vi "Agilent 33XXX Series Generate Modulated Waveform.vi"() -> ()   [LabVIEW 2010, in "AWG.lvlib"]
doc: "Shows how to configure and generate an amplitude modulated waveform."
uses:
  AWG.lvlib
  Agilent 33XXX Series.lvlib
  Public/Configure/Configure Modulation (Amplitude).vi
panel:
  in  "Serial Configuration":T1={"Baud Rate"=9600, "Parity"=0, "Data Bits"=8, "Flow Control"=4} {"Flow Control" items=["None", "XON/XOFF", "RTS/CTS", "XON/XOFF & RTS/CTS", "DTR/DSR", "XON/XOFF & DTR/DSR"]; "Data Bits" items=["7"=7, "8"=8]; "Parity" items=["None", "Odd", "Even", "Mark", "Space"]; "Baud Rate" items=["300"=300, "600"=600, "1200"=1200, "2400"=2400, "4800"=4800, "9600"=9600, "19200"=19200]}
  in  "DC Offset (0.00 V)":dbl
  in  "Amplitude (1 Vpp)":dbl=1.0
  in  "Waveform Function (1: Sine)":u16(ring)=1 items=["DC", "Sine", "Square", "Triangle", "Ramp", "Pulse", "Noise", "Sinc", "Negative Ramp", "Exponential Rise", "Exponential Fall", "Cardiac"]
  in  "Frequency (1000 Hz)":dbl=1000.0
  in  "Modulation Waveform (0: Sine)":i32(ring) items=["Sine", "Square", "Ramp", "Negative Ramp", "Triangle", "Noise", "Arbitrary Waveform"]
  in  "Amplitude Modulation Source (0: Internal)":i32(ring) items=["Internal", "External"]
  in  "Modulation Depth (100 %)":i32=100
  in  "Modulation Frequency (1000 Hz)":dbl=1000.0
  in  "VISA resource name":refnum<visa-resource-name>
  # "(c) 2005 - 2013 National Instruments.  ALL RIGHTS RESERVED."
  # "Carrier Settings"
  # "Modulation Settings"
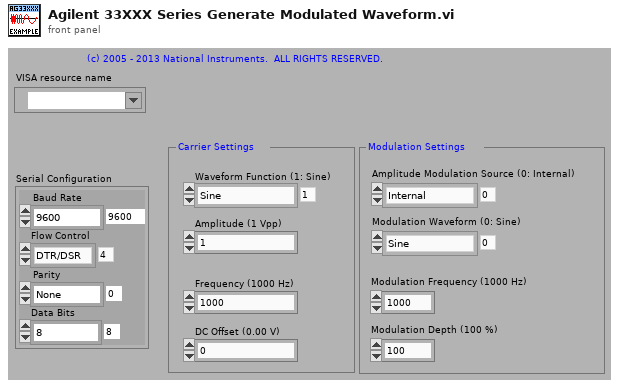
[diagram p1: front panel]
types:
  T1 = cluster{"Baud Rate":u32, "Parity":u16, "Data Bits":u16, "Flow Control":u16}
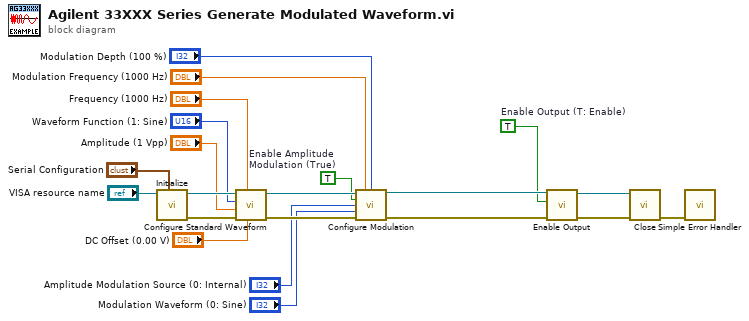
[diagram p0: block diagram]
diagram:
  w8 = TRUE  # Enable Output (T: Enable)
  w15 = TRUE  # Enable Amplitude Modulation (True)
  n1 = call "Initialize.vi"("Serial Configuration"="Serial Configuration", "VISA resource name"="VISA resource name") -> ("error out"=w20:errorcluster, "VISA resource name out"=w21:refnum<visa-resource-name>)  [unwired: 7 in, 1 out]
  n2 = call "Configure Standard Waveform.vi"("DC Offset (0.00 V)"="DC Offset (0.00 V)", "Frequency (1000 Hz)"="Frequency (1000 Hz)", "error in (no error)"=w20, "Amplitude (1)"="Amplitude (1 Vpp)", "Waveform Function (1: Sine)"="Waveform Function (1: Sine)", "VISA resource name"=w21) -> ("error out"=w18:errorcluster, "VISA resource name out"=w19:refnum<visa-resource-name>)  [unwired: 4 in]
  n3 = call-poly "Configure Modulation.vi"("VISA resource name"=w19, "Modulation Frequency (1000 Hz)"="Modulation Frequency (1000 Hz)", "Modulation Depth (100 %)"="Modulation Depth (100 %)", "Enable Amplitude Modulation (T: Enable)"=w15, "AM Source (0: Internal)"="Amplitude Modulation Source (0: Internal)", "Modulation Waveform (0: Sine)"="Modulation Waveform (0: Sine)", "error in (no error)"=w18) -> ("VISA resource name out"=w10:refnum<visa-resource-name>, "error out"=w9:errorcluster)  [unwired: 7 in]
  n4 = call "Enable Output.vi"("error in (no error)"=w9, "Enable Output  (T: Enable)"=w8, "VISA resource name"=w10) -> ("error out"=w4:errorcluster, "VISA resource name out"=w5:refnum<visa-resource-name>)  [unwired: 7 in]
  n5 = call "Close.vi"("error in (no error)"=w4, "VISA resource name"=w5) -> ("error out"=w16:errorcluster)  [unwired: 9 in]
  n6 = call <vilib>:"Simple Error Handler.vi"("error in (no error)"=w16) -> ()  [unwired: 4 in, 5 out]
